vi "setUp.vi"(8 "error in (no error)":errorcluster, 11 "reference in":refnum<class "TestTextFileSink.lvclass">) -> (0 "error out":errorcluster, 3 "reference out":refnum<class "TestTextFileSink.lvclass">)   [LabVIEW 2017, in "TestTextFileSink.lvclass"]
doc: "setUp runs prior to the test method during test execution. Use this method to initialize any object data required by your tests."
uses:
  TestTextFileSink.lvclass
  C:/Program Files (x86)/National Instruments/LabVIEW 2017/vi.lib/addons/_JKI Toolkits/VI Tester/TestCase.llb/TestCase.lvclass
  <vilib>/addons/_JKI Toolkits/VI Tester/TestCase.llb/TestCase.lvclass
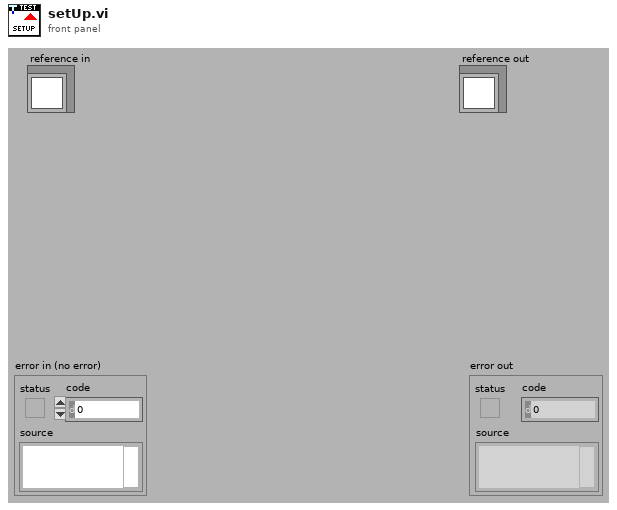
[diagram p1: front panel]
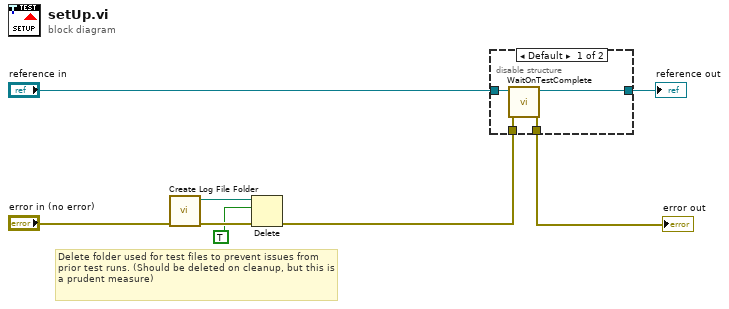
[diagram p0: block diagram]
diagram:
  # "Delete folder used for test files to prevent issues from prior test runs. (Should be deleted on cleanup, but this is a prudent measure)"
  n1 = call "Create Log File Folder.vi"("error in (no error)"="error in (no error)") -> ("error out"=w5:errorcluster, "Folder Path"=w6:path)  [unwired: 9 in]
  n2 = Delete(path (use dialog)=w6, entire hierarchy (F)=TRUE ("confirm (F)"), error in=w5) -> (error out=w1:errorcluster)  [unwired: 2 in, 2 out]
  n3 = disable-structure shown="Default" {
    disable-tunnel: w1 -> [w12 w13]
    disable-tunnel: [w11 w13] -> w8
    disable-tunnel: [w10 w14] -> w7
    disable-tunnel: "reference in" -> [w9 w14]
    frame condition #0 (active) {
      n4 = call <vilib>:"WaitOnTestComplete.vi"("error in (no error)"=w12, "TestCase in"=w9) -> ("error out"=w11:errorcluster, "TestCase out"=w10:refnum<class "TestTextFileSink.lvclass">)  [unwired: 8 in]
    }
    frame condition #1 {
    }
  }
  "error out" <- w8
  "reference out" <- w7
